vi "Auton Intake Dictation.vi"(7 "Roller Arms In":bool, 8 "First Iteration":bool, 9 "Roller Arms Same":bool, 10 "Time":dbl, 11 "Intake Select":dbl) -> (3 "Time has Elapsed":bool)   [LabVIEW 2014]
uses:
  Begin/Global Variables.vi
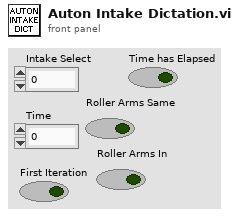
[diagram p1: front panel]
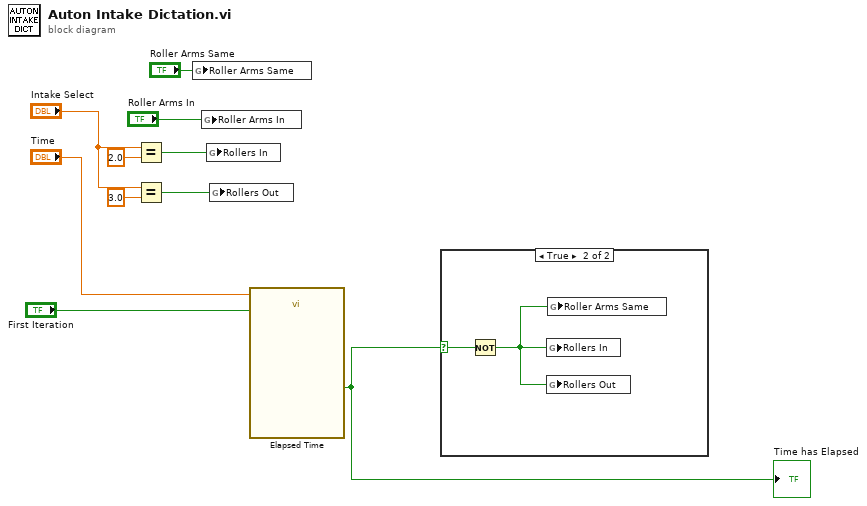
[diagram p0: block diagram]
diagram:
  n1 = Equal?(x="Intake Select", y=2.0) -> (x = y?=w7:bool)
  n2 = Equal?(x="Intake Select", y=3.0) -> (x = y?=w6:bool)
  n3 = global write "Global Variables.vi" "Roller Arms Same"("Roller Arms Same") -> ()
  n4 = global write "Global Variables.vi" "Roller Arms In"("Roller Arms In") -> ()
  n5 = global write "Global Variables.vi" "Rollers In"(w7) -> ()
  n6 = global write "Global Variables.vi" "Rollers Out"(w6) -> ()
  n7 = call "Elapsed Time"("Time Target (s)"="Time", "Reset"="First Iteration") -> ("Time has Elapsed"=w9:bool)  [unwired: 10 in, 7 out]
  "Time has Elapsed" <- w9
  n8 = case shown="True" w9 {
    selector: w9 -> [_ w12]
    frame False {
    }
    frame True {
      n9 = Not(x=w12) -> (.not. x?=w11:bool)
      n10 = global write "Global Variables.vi" "Rollers In"(w11) -> ()
      n11 = global write "Global Variables.vi" "Rollers Out"(w11) -> ()
      n12 = global write "Global Variables.vi" "Roller Arms Same"(w11) -> ()
    }
  }
